vi "HeaderAction.vi"(0 "InstrClass":refnum<class "E8267D.lvclass"> caption="DNL_LabVIEW Object in", 11 "error in (no error)":errorcluster caption="entrée d'erreur (pas d'erreur)") -> (4 "InstrClassOut":refnum<class "E8267D.lvclass"> caption="DNL_LabVIEW Object out", 6 "DataNames":string[](array[string]), 8 "Instr Name":string, 10 "HeaderString":string, 13 "ArrDisplayNames":string[](array[string]), 14 "DisplayNames":string[](array[string]), 15 "error out":errorcluster caption="sortie d'erreur")   [LabVIEW 2019, in "E8267D.lvclass"]
uses:
  E8267D.lvclass
  C:/Programmes Labview/LabscanV1A/DevicesClass/BaseDevice/BaseDevice.lvclass
  E8267D.lvclass/E8267D.ctl
  BaseDevice/BaseDevice.lvclass
panel:
  in  "FUnits":u16(ring) caption="Units" items=["Hz", "MHz", "GHz"]
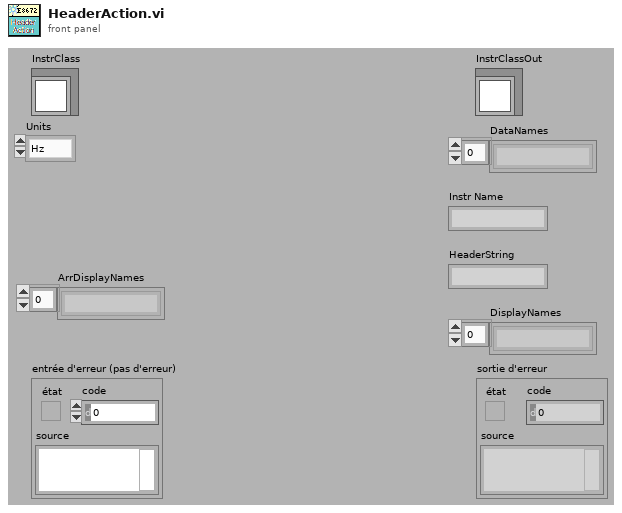
[diagram p1: front panel]
types:
  T1 = typedef "E8267D.lvclass/E8267D_Func.ctl" = enum16{"SetPower (dBm)", "SetFrequency (Hz)"}
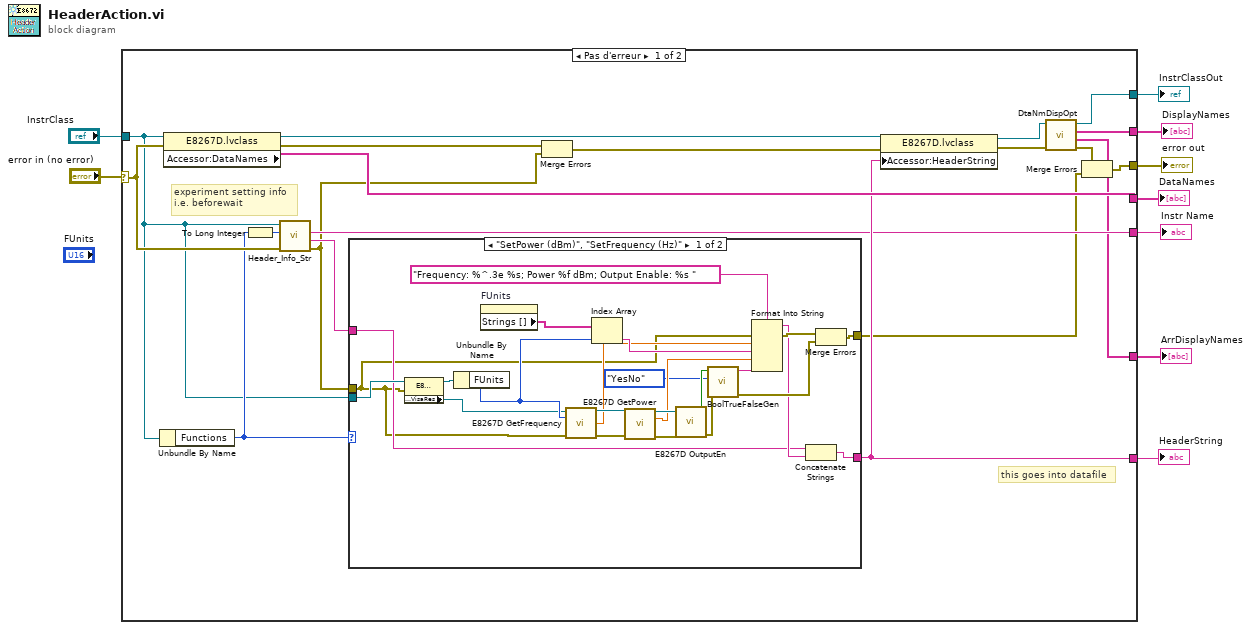
[diagram p0: block diagram]
diagram:
  n1 = case shown="Pas d'erreur" "error in (no error)" {
    selector: "error in (no error)" -> [w18 w56]
    tunnel: [w26 _] -> w8
    tunnel: [w29 _] -> w7
    tunnel: "InstrClass" -> [w13 w57]
    tunnel: [w11 w56] -> w5
    tunnel: [w23 w57] -> w3
    tunnel: [w20 _] -> w4
    tunnel: [w21 _] -> w2
    tunnel: [w14 _] -> w1
    frame No Error {
      # "this goes into datafile"
      # "experiment setting info\ni.e. beforewait"
      n2 = Unbundle By Name(w13) -> ("Functions"=w16:T1)
      n3 = property class="E8267D.lvclass"(reference=w13, error in=w18) -> (reference out=w28:refnum<class "E8267D.lvclass">, error out=w27:errorcluster, "Accessor:DataNames"=w29:string[])
      n4 = To Long Integer(number=w16) -> (32bit integer=w15:i32)
      n5 = call-dynamic "Header_Info_Str.vi"("error in (no error)"=w18, "Functions"=w15, "DefaultDev in"=w13) -> ("error out"=w12:errorcluster, "HdrInfoStr"=w19:string, "InstrumentName"=w20:string)  [unwired: 5 in, 1 out]
      n6 = case shown="\"SetPower (dBm)\", \"SetFrequency (Hz)\"" w16 {
        tunnel: [w33 w55] -> w26
        tunnel: w19 -> [w32 w55]
        tunnel: w13 -> [w48 _]
        tunnel: w12 -> [w31 w54]
        tunnel: [w36 w54] -> w10
        frame "SetPower (dBm)", "SetFrequency (Hz)" {
          n7 = property class="E8267D.lvclass"(reference=w48, error in=w31) -> (reference out=w49:refnum<class "E8267D.lvclass">, "Accessor:VisaRes"=w30:refnum<visa-resource-name>)  [unwired: 1 out]
          n8 = Unbundle By Name(w49) -> ("FUnits"=w46:u16)
          n9 = property on="FUnits" class="MDér (strict)"() -> ("Strings []"=w47:string[])  [unwired: 2 in, 2 out]
          n10 = call <userlib>:"E8267D GetFrequency.vi"("VISA Rsrc"=w30, "FUnits"=w46, "error in (no error)"=w31) -> ("VISA Rsrc Out"=w52:refnum<visa-resource-name>, "Frequency (Units)"=w43:dbl, "error out"=w53:errorcluster)  [unwired: 9 in, 1 out]
          n11 = Index Array(array=w47, index=w46) -> (element=w44:string)
          n12 = call <userlib>:"E8267D GetPower.vi"("VISA Rsrc"=w52, "error in (no error)"=w53) -> ("VISA Rsrc Out"=w50:refnum<visa-resource-name>, "Power (dBm)"=w42:dbl, "error out"=w51:errorcluster)  [unwired: 11 in]
          n13 = call <userlib>:"E8267D OutputEn.vi"("VISA Rsrc"=w50, "error in (no error)"=w51) -> ("Enabled"=w41:bool, "error out"=w40:errorcluster)  [unwired: 11 in, 1 out]
          n14 = call <userlib>:"BoolTrueFalseGen.vi"("Error in"=w40, "Énum"=enum16{"TrueFalse", "YesNo", "OnOff"}."YesNo", "Bool"=w41) -> ("Error out"=w35:errorcluster, "TrueFalse"=w39:string)  [unwired: 6 in]
          n15 = Format Into String(format string="Frequency: %^.3e %s; Power %f dBm; Output Enable: %s " ("chaîne de format"), error in=w31, w43, w44, w42, w39) -> (resulting string=w34:string, error out=w37:errorcluster)  [unwired: 1 in]
          n16 = Concatenate Strings(w32, w34) -> (w33:string)
          n17 = Merge Errors(w37, w35) -> (w36:errorcluster)
        }
        frame Default {
        }
      }
      n18 = Merge Errors(w27, w12) -> (w17:errorcluster)
      n19 = property class="E8267D.lvclass"(reference=w28, error in=w17, "Accessor:HeaderString"=w26) -> (reference out=w22:refnum<class "E8267D.lvclass">, error out=w25:errorcluster)
      n20 = call "DtaNmDispOpt.vi"("error in (no error)"=w25, "BaseDevice en entrée"=w22) -> ("error out"=w24:errorcluster, "ArrDisplayNames"=w14:string[], "DisplayNames"=w21:string[], "BaseDevice en sortie"=w23:refnum<class "E8267D.lvclass">)  [unwired: 6 in]
      n21 = Merge Errors(w24, w10) -> (w11:errorcluster)
    }
    frame Error {
    }
  }
  "error out" <- w5
  "InstrClassOut" <- w3
  "DataNames" <- w7
  "HeaderString" <- w8
  "Instr Name" <- w4
  "DisplayNames" <- w2
  "ArrDisplayNames" <- w1
